vi "ALTS-2015 Check DI for Station Enable.vi"(8 "error in":errorcluster, 11 "DI Index":i32) -> (0 "error out":errorcluster, 3 "Station Enable?":bool)   [LabVIEW 2013]
doc: "Copyright © 2005, Soliton Technologies.\nAll rights reserved."
uses:
  SLL DAQ Engine/Software/Source Code/Sub VIs/DAQ Engine/Controls/SLL DE List of Digital Inputs.ctl
  Controls/ALTS-2015 Station Cluster.ctl
  Controls/ALTS-2015 LV2GBL Options.ctl
panel:
  in  "Station Enum":T1
  in  "List of Digital Inputs":T2
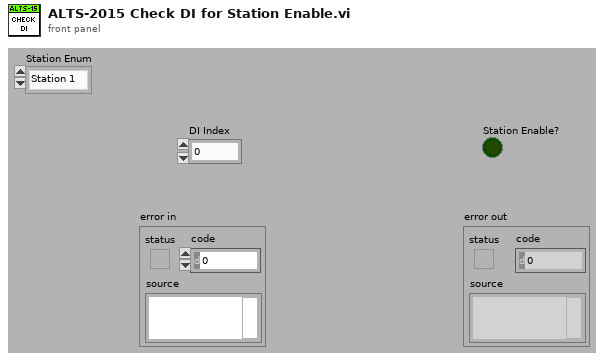
[diagram p1: front panel]
types:
  T1 = typedef "ALTS-2015 Station Cluster.ctl" = enum16{"Station 1", "Station 2", "Station 3", "Station 4"}
  T2 = typedef "SLL DE List of Digital Inputs.ctl" = enum16{"STATION1_START", "STATION1_STOP", "STATION1_CLAMPED", "STATION1_TC_PASS", "STATION1_TC_FAIL", "STATION1_TTA", "STATION1_TTB", "STATION2_START", "STATION2_STOP", "STATION2_CLAMPED", "STATION2_TC_PASS", "STATION2_TC_FAIL", "STATION2_TTA", "STATION2_TTB", "STATION3_START", "STATION3_STOP", "STATION3_CLAMPED", "STATION3_TC_PASS", "STATION3_TC_FAIL", "STATION3_TTA", "STATION3_TTB", "STATION4_START", "STATION4_STOP", "STATION4_CLAMPED", "STATION4_TC_PASS", "STATION4_TC_FAIL", "STATION4_TTA", "STATION4_TTB"}
  T3 = typedef "ALTS-2015 LV2GBL Options.ctl" = enum16{"Read all", "Write all"}
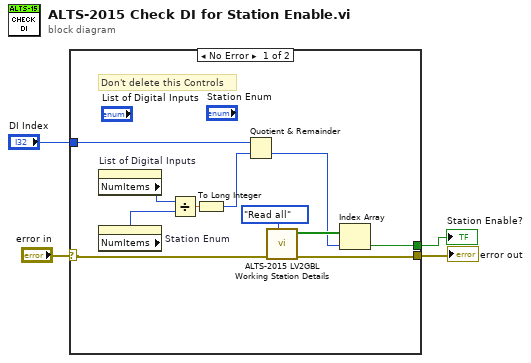
[diagram p0: block diagram]
diagram:
  n1 = case shown="No Error" "error in" {
    selector: "error in" -> [w14 w17]
    tunnel: [w12 w17] -> w3
    tunnel: "DI Index" -> [w11 _]
    tunnel: [w8 FALSE ("Station4 Enable")] -> w1
    frame No Error {
      # "Don't delete this Controls"
      n2 = property on="List of Digital Inputs" class="Enum (strict)"() -> ("NumItems"=w7:u32)  [unwired: 2 in, 2 out]
      n3 = property on="Station Enum" class="Enum (strict)"() -> ("NumItems"=w6:u32)  [unwired: 2 in, 2 out]
      n4 = Divide(x=w7, y=w6) -> (x/y=w5:dbl)
      n5 = To Long Integer(number=w5) -> (32bit integer=w10:i32)
      n6 = Quotient & Remainder(x=w11, y=w10) -> (floor(x/y)=w9:i32)  [unwired: 1 out]
      n7 = call "ALTS-2015 LV2GBL Working Station Details.vi"("Options"=ALTS-2015_LV2GBL_Options."Read all", "error in"=w14) -> ("error out"=w12:errorcluster, "Station  Enable Array"=w13:bool[])  [unwired: 8 in]
      n8 = Index Array(array=w13, index=w9) -> (element=w8:bool)
    }
    frame Error {
    }
  }
  "error out" <- w3
  "Station Enable?" <- w1
